vi "splashScreen.vi"() -> ()   [LabVIEW 2014]
panel:
  in  "error in (no error)":errorcluster
  out "error out":errorcluster
  # "Testando a splashScreen"
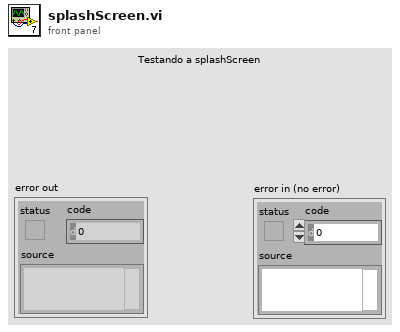
[diagram p1: front panel]
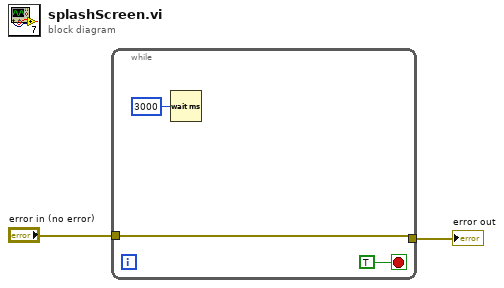
[diagram p0: block diagram]
diagram:
  n1 = while {
    tunnel: "error in (no error)" -> [w3]
    tunnel: [w3] -> w1
    stop <- TRUE stop-if-true
    n2 = Wait (ms)(milliseconds to wait=u32 3000) -> ()  [unwired: 1 out]
  }
  "error out" <- w1
